vi "G#ModifyAttributeDiagramTemplate.vi"   [LabVIEW 2020]
doc: "This is a G# modify attribute DVR structure. Paste this in your diagram together with the .._GetAttributes to modify the attributes (replace attribute ref and error constant)."
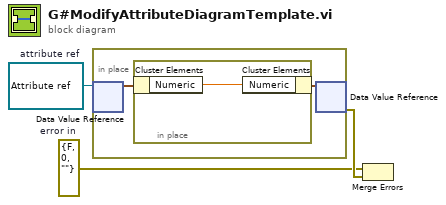
[diagram p0: block diagram]
diagram:
  w1 = errorcluster {"status"=FALSE, "code"=0, "source"=""}  # error in
  w2 = refnum<data-value> refnum  # attribute ref
  n1 = in-place {
    n2 = in-place-dvr #1(w2) -> (w4:cluster{"Numeric":dbl})  [unwired: 1 out]
    n3 = in-place {
      n4 = in-place-cluster #2(w4) -> ("Numeric"=w6:dbl)
      n5 = in-place-cluster #2("Numeric"=w6) -> (w5:cluster{"Numeric":dbl})
    }
    n6 = in-place-dvr #1(w5) -> (w3:errorcluster)  [unwired: 1 out]
  }
  n7 = Merge Errors(w1, w3) -> ()  [unwired: 1 out]
